vi "test_libssh2_userauth_publickey.vi"() -> ()   [LabVIEW 2017, in "integration_tests.lvlib"]
uses:
  integration_tests.lvlib
  libssh2/libssh2_session_handshake_tcp.vi
  libssh2/libssh2_init_default.vi
  libssh2/libssh2_session_init_ex.vi
  <vilib>/Utility/tcp.llb/TCP Get Raw Net Object.vi
  libssh2/libssh2_session_handshake_socket.vi
  support/callback_userauth_publickey_sign_function.vi
  libssh2/libssh2.lvlib
  support/support.lvlib
  <vilib>/PNR/Transparent Assertions/Transparent Assertions/Transparent Assertions.lvlib
panel:
  out "error out":errorcluster
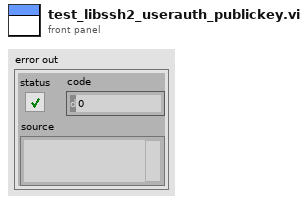
[diagram p1: front panel]
types:
  T1 = typedef "libssh2.lvlib/Session Refnum.ctl" = refnum<k1>
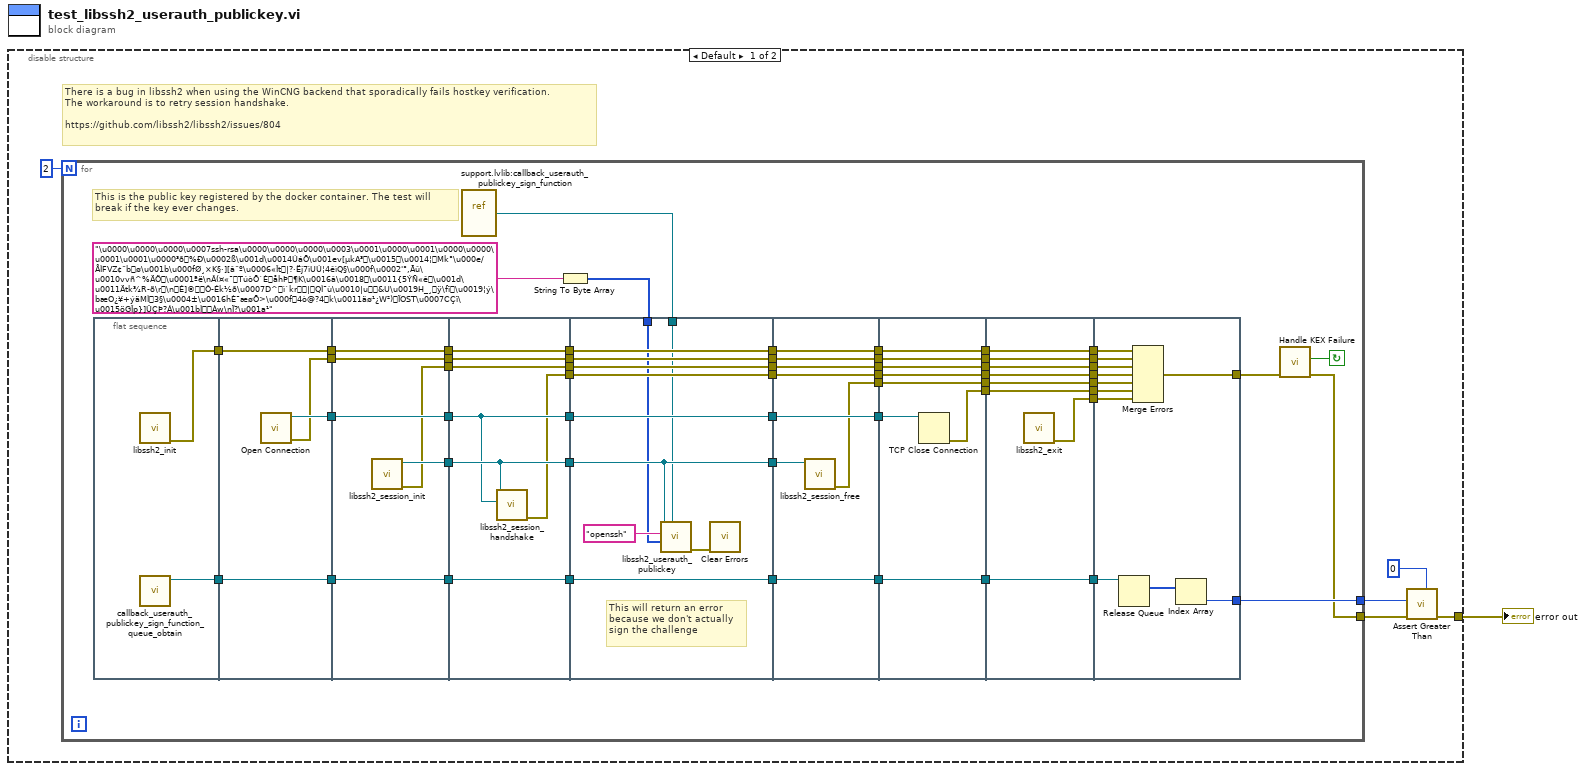
[diagram p0: block diagram]
diagram:
  n1 = disable-structure shown="Default" {
    disable-tunnel: [w6 _] -> w1
    frame condition #0 (active) {
      # "There is a bug in libssh2 when using the WinCNG backend that sporadically fails hostkey verification.\nThe workaround is to retry session handshake.\n\nhttps://github.com/libssh2/libssh2/issues/804"
      n2 = for {
        N: 2 -> [_]
        tunnel: [w10] -> w2
        tunnel: [w7] -> w5
        stop <- w8 continue-if-true
        # "This is the public key registered by the docker container. The test will\nbreak if the key ever changes."
        n3 = flat-sequence {
          tunnel: [w63] -> w61
          tunnel: [w62] -> w60
          tunnel: [w67] -> w59
          tunnel: w61 -> [w66]
          tunnel: [w66] -> w58
          tunnel: [w65] -> w57
          tunnel: [w64] -> w56
          tunnel: w60 -> [w64]
          tunnel: w59 -> [w73]
          tunnel: [w73] -> w55
          tunnel: w58 -> [w72]
          tunnel: [w72] -> w54
          tunnel: w57 -> [w71]
          tunnel: [w71] -> w53
          tunnel: [w70] -> w52
          tunnel: [w69] -> w51
          tunnel: [w68] -> w50
          tunnel: w56 -> [w68]
          tunnel: w55 -> [w76]
          tunnel: [w76] -> w49
          tunnel: w54 -> [w80]
          tunnel: [w80] -> w48
          tunnel: w53 -> [w79]
          tunnel: [w79] -> w47
          tunnel: [w78] -> w46
          tunnel: w52 -> [w78]
          tunnel: w51 -> [w77]
          tunnel: [w77] -> w45
          tunnel: [w75] -> w44
          tunnel: [w74] -> w43
          tunnel: w50 -> [w74]
          tunnel: w49 -> [w91]
          tunnel: [w91] -> w42
          tunnel: w48 -> [w90]
          tunnel: [w90] -> w41
          tunnel: w47 -> [w89]
          tunnel: [w89] -> w40
          tunnel: w46 -> [w86]
          tunnel: w45 -> [w88]
          tunnel: [w88] -> w39
          tunnel: w44 -> [w87]
          tunnel: [w87] -> w38
          tunnel: [w86] -> w37
          tunnel: w13 -> [w84]
          tunnel: w11 -> [w83]
          tunnel: [w82] -> w36
          tunnel: w43 -> [w82]
          tunnel: w42 -> [w99]
          tunnel: [w99] -> w35
          tunnel: w41 -> [w98]
          tunnel: [w98] -> w34
          tunnel: w40 -> [w97]
          tunnel: [w97] -> w33
          tunnel: w39 -> [w96]
          tunnel: [w96] -> w32
          tunnel: w38 -> [w95]
          tunnel: [w95] -> w31
          tunnel: [w94] -> w30
          tunnel: w37 -> [w93]
          tunnel: [w92] -> w29
          tunnel: w36 -> [w92]
          tunnel: w35 -> [w107]
          tunnel: w34 -> [w106]
          tunnel: [w106] -> w28
          tunnel: w33 -> [w105]
          tunnel: [w105] -> w27
          tunnel: [w104] -> w26
          tunnel: w32 -> [w103]
          tunnel: [w103] -> w25
          tunnel: w31 -> [w102]
          tunnel: [w102] -> w24
          tunnel: [w101] -> w23
          tunnel: w30 -> [w101]
          tunnel: [w100] -> w22
          tunnel: w29 -> [w100]
          tunnel: w28 -> [w115]
          tunnel: [w115] -> w21
          tunnel: w27 -> [w114]
          tunnel: [w114] -> w20
          tunnel: w26 -> [w113]
          tunnel: [w113] -> w19
          tunnel: [w112] -> w18
          tunnel: w25 -> [w111]
          tunnel: [w111] -> w17
          tunnel: w24 -> [w110]
          tunnel: [w110] -> w16
          tunnel: [w109] -> w15
          tunnel: w23 -> [w109]
          tunnel: [w108] -> w14
          tunnel: w22 -> [w108]
          tunnel: w21 -> [w126]
          tunnel: w20 -> [w125]
          tunnel: w19 -> [w124]
          tunnel: w18 -> [w123]
          tunnel: w17 -> [w122]
          tunnel: w16 -> [w121]
          tunnel: w15 -> [w120]
          tunnel: w14 -> [w118]
          tunnel: [w117] -> w10
          tunnel: [w116] -> w9
          frame #0 {
            n4 = call-poly "libssh2_init.vi"() -> ("error out"=w63:errorcluster)  [unwired: 11 in]
            n5 = call "callback_userauth_publickey_sign_function_queue_obtain.vi"() -> ("queue out"=w62:refnum<queue>)  [unwired: 10 in, 1 out]
          }
          frame #1 {
            n6 = call "Open Connection.vi"() -> ("error out"=w65:errorcluster, "connection ID"=w67:refnum<k5>)  [unwired: 10 in]
          }
          frame #2 {
            n7 = call "libssh2_session_init.vi"() -> ("error out"=w69:errorcluster, "session"=w70:T1)  [unwired: 10 in]
          }
          frame #3 {
            n8 = call-poly "libssh2_session_handshake.vi"("tcp connection"=w76, "session"=w78) -> ("error out"=w75:errorcluster)  [unwired: 9 in]
          }
          frame #4 {
            # "This will return an error\nbecause we don't actually\nsign the challenge"
            n9 = call "libssh2_userauth_publickey.vi"("sign"=w84, "public key data"=w83, "username"="openssh", "session"=w86) -> ("error out"=w81:errorcluster)  [unwired: 7 in]
            n10 = call <vilib>:"Clear Errors.vi"("error in (no error)"=w81) -> ()  [unwired: 5 in, 2 out]
          }
          frame #5 {
            n11 = call "libssh2_session_free.vi"("session"=w93) -> ("error out"=w94:errorcluster)  [unwired: 10 in]
          }
          frame #6 {
            n12 = TCP Close Connection(connection ID=w107) -> (error out=w104:errorcluster)  [unwired: 2 in, 1 out]
          }
          frame #7 {
            n13 = call "libssh2_exit.vi"() -> ("error out"=w112:errorcluster)  [unwired: 11 in]
          }
          frame #8 {
            n14 = Release Queue(queue=w118) -> (remaining elements=w119:i64[])  [unwired: 2 in, 2 out]
            n15 = Merge Errors(w126, w125, w122, w121, w120, w124, w123) -> (w116:errorcluster)
            n16 = Index Array(array=w119) -> (element=w117:i64)  [unwired: 1 in]
          }
        }
        n17 = vi-ref "support.lvlib:callback_userauth_publickey_sign_function.vi"() -> (w13:refnum<vi>)
        n18 = String To Byte Array(string="\u0000\u0000\u0000\u0007ssh-rsa\u0000\u0000\u0000\u0003\u0001\u0000\u0001\u0000\u0000\u0001\u0001\u0000³ð%Ð\u0002ß\u001d\u0014ÚáÕ\u001ev[µkA³\u0015\u0014¦Mk°\u000e/ÅÌFVZ¢¨bø\u001b\u000fØ¸×K§·][â¨º\u0006«Ît|?·Ëj7ìUÚ¦4êìQ§\u000f\u0002'°,Ãû\u0010vvñ^%ÄÖ\u0001ªë\nÂ(¤«¯TúòÕ`ÈåhÞ¶K\u0016â\u0018\u0011{5ÝÑ«ê\u001d\u0011Ätk¾R­õ\r\nÉ]©Ô-Ék½ð\u0007D^ì`kr|QÌ¯ù\u0010|u&U\u0019H_¸ÿ\fï\u0019¦ý\bæO¿¥+ýäMÌ3§\u0004±\u0016hÈ¯æøÕ>\u000f4ò@?4k\u0011äø¹¿W²)ÏOST\u0007CÇï\u0015öGÎp}]ÛÇÞ?Á\u001bÌÀw\nÏ?\u001a¹") -> (unsigned byte array=w11:u8[])
        n19 = call "Handle KEX Failure.vi"("error in (no error)"=w9) -> ("error out"=w7:errorcluster, "KEX Failure"=w8:bool)  [unwired: 9 in]
      }
      n20 = call <vilib>:"Assert Greater Than.vi"("Expected"=i64 0 ("element"), "error in (no error)"=w5, "Actual"=w2) -> ("error out"=w6:errorcluster)  [unwired: 8 in]
    }
    frame condition #1 {
    }
  }
  "error out" <- w1
